vi "Light_Power_Reading.vi"() -> (0 "DAQ Error":errorcluster)   [LabVIEW 2017]
uses:
  Globals/Meas_global.vi
panel:
  out "Waveform Graph":dbl[][](graph)
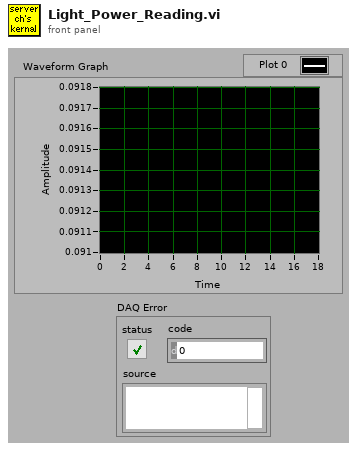
[diagram p1: front panel]
types:
  T1 = typedef "Analysis_info_cluster.ctl" = cluster{"Colour":u32, "Inst type":T2, "Inst name":string, "Symbol":string, "Code name":string, "Extra Info":string, "Inst Array":T3, "Extra Titles":string[], "Extra Values":string[], "U":dbl, "u^2":dbl, "u^3":dbl, "u^4":dbl, "Skew_u":dbl, "Kurt_u":dbl, "Sd Error in Mean":dbl, "% u'/U":dbl, "X":dbl, "Y":dbl, "Z":dbl, "Timescale integral Estimate":dbl, "Sd Error in Variance":dbl, "Calib File":path, "Calib Constants":dbl[], "Output Position":bool, "Full Stats":bool, "Av Sampling Rate":dbl, "Av No of Samples":dbl, "Total Meas Time (s)":dbl, "ADAM Ch Name":string, "Max value":dbl, "Min value":dbl, "Sync Delay Time (s)":dbl}
  T2 = typedef "Inst_type.ctl" = enum16{"Propeller anemometer", "Raw voltage", "Pressure Transducer", "Pitot-static tube", "Preston tube", "Hot wire", "Cross wire 1", "Cross wire 2", "Generic Linear", "Generic Polynomial", "Generic BackPoly", "Fast FID", "Thermocouple", "Cold wire", "Pulsed Wire", "LDA Vel", "LDA Tran time", "LDA Arr time", "Microphone"}
  T3 = typedef "Instrument_Array.ctl" = enum16{"PWA", "LDA", "Analogue"}
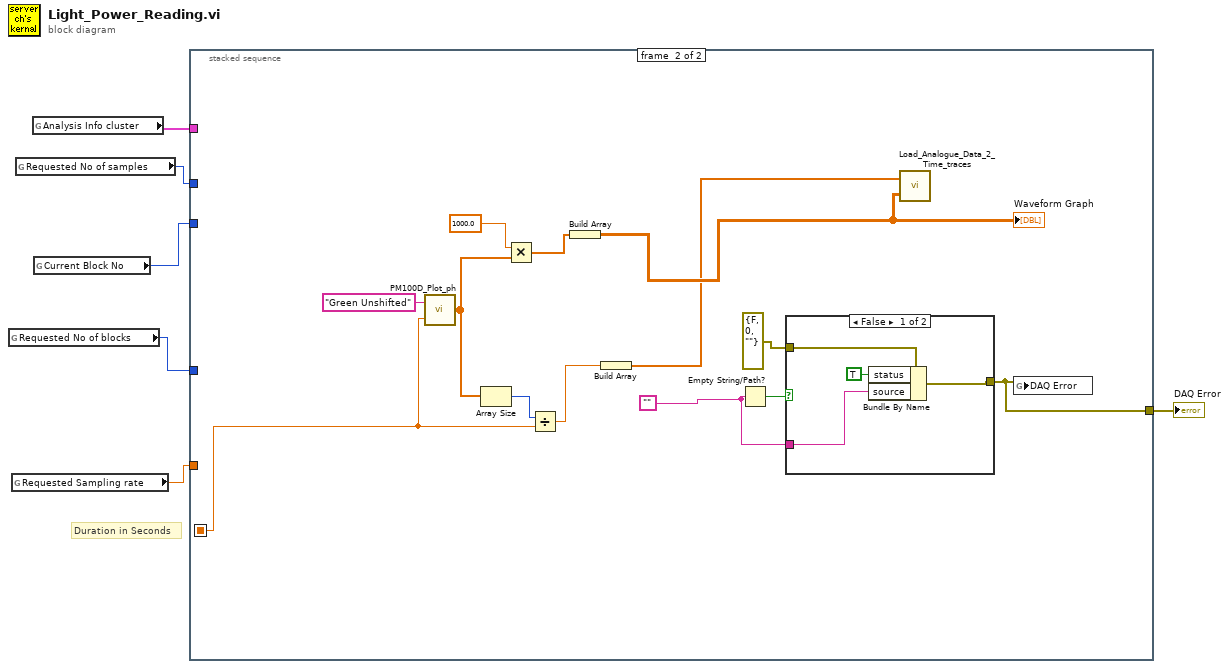
[diagram p0: block diagram]
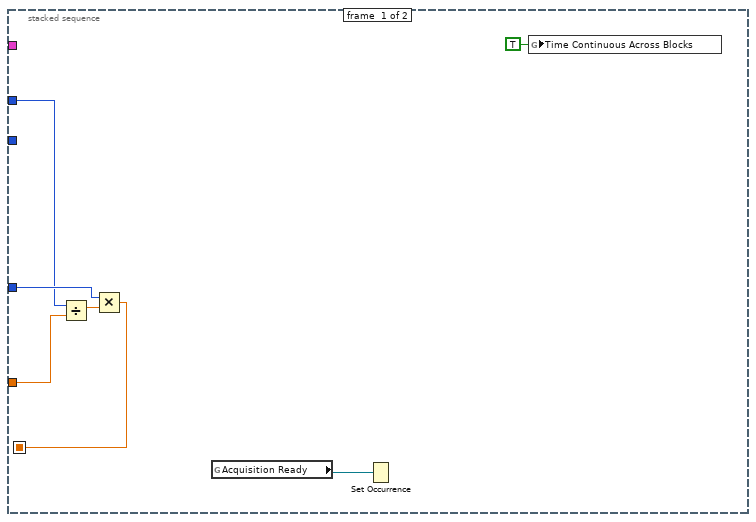
[diagram p2: hidden frame]
diagram:
  # "Duration in Seconds"
  n1 = global read "Meas_global.vi" "Requested No of blocks"() -> (w2:i32)
  n2 = global read "Meas_global.vi" "Requested Sampling rate"() -> (w5:dbl)
  n3 = global read "Meas_global.vi" "Requested No of samples"() -> (w6:i32)
  n4 = global read "Meas_global.vi" "Analysis Info cluster"() -> (w3:T1[])
  n5 = global read "Meas_global.vi" "Current Block No"() -> (w4:i32)
  n6 = stacked-sequence {
    seq-local: [w10 _] -> [_ w20]
    tunnel: w6 -> [w9 _]
    tunnel: w4 -> [_ _]
    tunnel: w3 -> [_ _]
    tunnel: w5 -> [w13 _]
    tunnel: w2 -> [w11 _]
    tunnel: [_ w23] -> w1
    frame #0 {
      n7 = Divide(x=w9, y=w13) -> (x/y=w12:dbl)
      n8 = Multiply(x=w11, y=w12) -> (x*y=w10:dbl)
      n9 = global read "Meas_global.vi" "Acquisition Ready"() -> (w7:refnum<k4>)
      n10 = Set Occurrence(w7) -> ()
      n11 = global write "Meas_global.vi" "Time Continuous Across Blocks"(TRUE ("Time Continuous across Blocks")) -> ()
    }
    frame #1 {
      w24 = ""
      n12 = call "PM100D_Plot_ph.vi"("Meas Time (s)"=w20, "Beam Name"="Green Unshifted") -> ("Array"=w19:dbl[])
      n13 = Array Size(array=w19) -> (size(s)=w21:i32)
      n14 = Multiply(x=1000.0, y=w19) -> (x*y=w17:dbl[])
      n15 = Divide(x=w21, y=w20) -> (x/y=w15:dbl)
      n16 = Build Array(w17) -> (w16:dbl[][])
      "Waveform Graph" <- w16
      n17 = Build Array(w15) -> (w14:dbl[])
      n18 = Empty String/Path?(string/path=w24) -> (empty?=w26:bool)
      n19 = case shown="False" w26 {
        tunnel: errorcluster {"status"=FALSE, "code"=0, "source"=""} ("DAQ Error") -> [w30 w31]
        tunnel: [w29 w31] -> w23
        tunnel: w24 -> [w27 _]
        frame False {
          n20 = Bundle By Name(cluster=w30, "status"=TRUE, "source"=w27) -> (w29:errorcluster)
        }
        frame True {
        }
      }
      n21 = call "Load_Analogue_Data_2_Time_traces.vi"("Voltage Array"=w16, "Sampling Rate (Hz)"=w14) -> ()  [unwired: 1 in]
      n22 = global write "Meas_global.vi" "DAQ Error"(w23) -> ()
    }
  }
  "DAQ Error" <- w1
